vi "Test the mean filter.vi"() -> ()   [LabVIEW 2016]
panel:
  out "Array 2":i32[](array[numeric])
  out "Array":i32[](array[numeric])
  out "Mean false":i32
  out "Mean true":i32
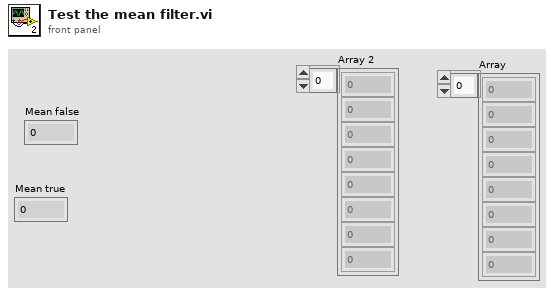
[diagram p1: front panel]
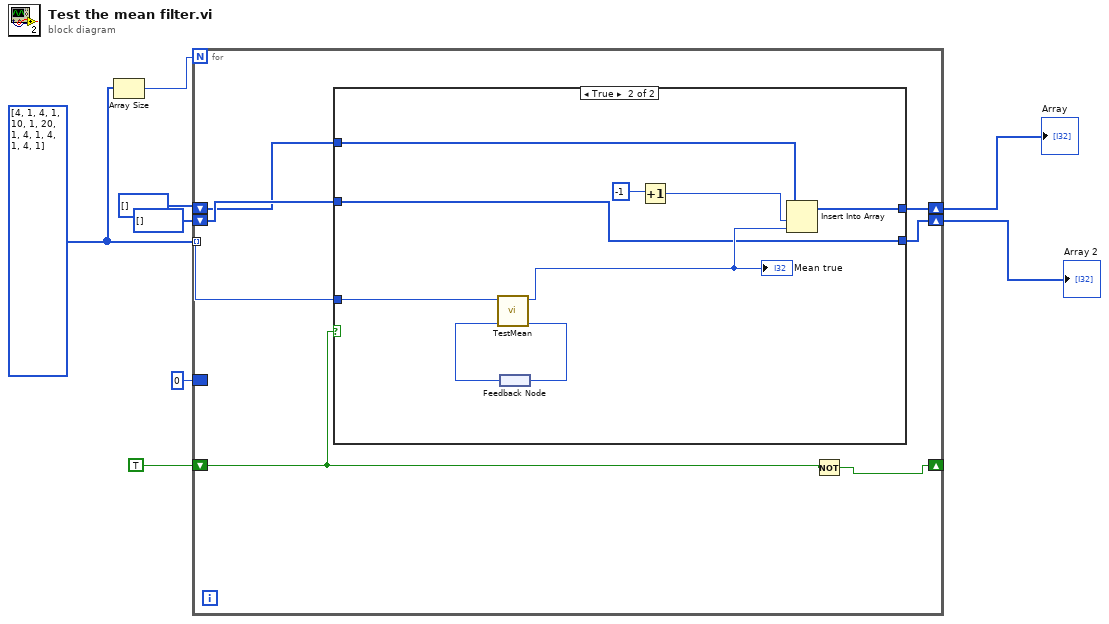
[diagram p0: block diagram]
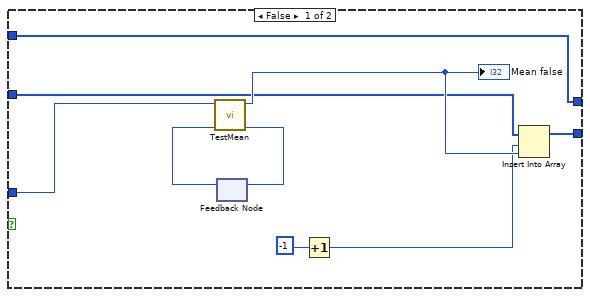
[diagram p2: hidden frame]
diagram:
  w7 = i32[] [4, 1, 4, 1, 10, 1, 20, 1, 4, 1, 4, 1, 4, 1]
  n1 = Array Size(array=w7) -> (size(s)=w6:i32)
  n2 = for {
    N: w6 -> [_]
    tunnel: w7 -> [w15] mode=indexing
    shift-right: [w14] -> _
    shift-left: TRUE -> [w13]
    border: 0 ("x+y") -> [_]
    shift-right: [w12] -> w1
    shift-left: i32[] [] -> [w11]
    shift-right: [w10] -> w2
    shift-left: i32[] [] -> [w9]
    n3 = case shown="True" w13 {
      tunnel: w15 -> [w22 w33]
      tunnel: [w18 w27] -> w12
      tunnel: w11 -> [w17 w27]
      tunnel: [w16 w26] -> w10
      tunnel: w9 -> [w16 w25]
      frame False {
        n4 = feedback #1() -> (w23:i32)  [unwired: 1 in]
        n5 = call "TestMean.vi"("x"=w23, "Numeric"=w22) -> ("x+y"=w24:i32, "Mean"=w21:i32)  [unwired: 8 in]
        "Mean false" <- w21
        n6 = feedback-in #1(w24) -> ()
        n7 = Increment(x=-1) -> (x+1=w20:i32)
        n8 = Insert Into Array(array=w17, index=w20, new element=w21) -> (w18:i32[])
      }
      frame True {
        n9 = feedback #2() -> (w31:i32)
        n10 = call "TestMean.vi"("x"=w31, "Numeric"=w33) -> ("x+y"=w32:i32, "Mean"=w30:i32)  [unwired: 8 in]
        "Mean true" <- w30
        n11 = feedback-in #2(w32) -> ()
        n12 = Increment(x=-1) -> (x+1=w29:i32)
        n13 = Insert Into Array(array=w25, index=w29, new element=w30) -> (w26:i32[])
      }
    }
    n14 = Not(x=w13) -> (.not. x?=w14:bool)
  }
  "Array" <- w2
  "Array 2" <- w1
